vi "tm_getcaptureinfo_40.vi"(8 "error in (no error)":errorcluster, 11 "Handle in":u32) -> (0 "error out":errorcluster, 1 "Frame Count":i32, 2 "Frame Index":i32, 3 "Handle out":u32)   [LabVIEW 2023]
uses:
  tmcamcon.dll
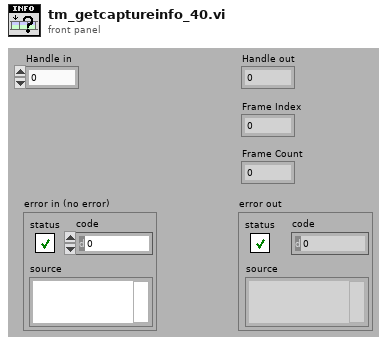
[diagram p1: front panel]
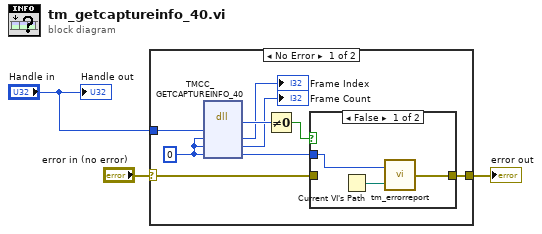
[diagram p0: block diagram]
diagram:
  n1 = case shown="No Error" "error in (no error)" {
    selector: "error in (no error)" -> [w8 w17]
    tunnel: [w7 w17] -> w2
    tunnel: "Handle in" -> [w11 _]
    frame No Error {
      w4 = 0 ("Erval")
      n2 = dll-call lib="tmcamcon.dll" fn="TMCC_GETCAPTUREINFO_40"("HDCAM"=w11, "frameindex"=w4, "framecount"=w4, "Erval"=w4) -> ("return type"=w12:u32, "frameindex"=→"Frame Index":i32, "framecount"=→"Frame Count":i32, "Erval"=w6:i32)  [unwired: 4 in, 2 out]
      n3 = Not Equal To 0?(x=w12) -> (x != 0?=w5:bool)
      n4 = case shown="False" w5 {
        tunnel: w8 -> [_ w16]
        tunnel: [w14 w16] -> w7
        tunnel: w6 -> [w13 _]
        frame False {
          n5 = Current VI's Path() -> (path=w15:path)
          n6 = call "tm_errorreport.vi"("Source"=w15, "Error"=w13) -> ("error out"=w14:errorcluster)
        }
        frame True {
        }
      }
    }
    frame Error {
    }
  }
  "error out" <- w2
  "Handle out" <- "Handle in"
